vi "Is Connected.vi"(8 "error in (no error)":errorcluster, 11 "FileStream in":refnum<class "FileStream.lvclass">) -> (0 "error out":errorcluster, 2 "Connected":bool, 3 "FileStream out":refnum<class "FileStream.lvclass">)   [LabVIEW 2020, in "Stream.lvlib" / "FileStream.lvclass"]
uses:
  FileStream.lvclass
  FileStream.lvclass/FileStream.ctl
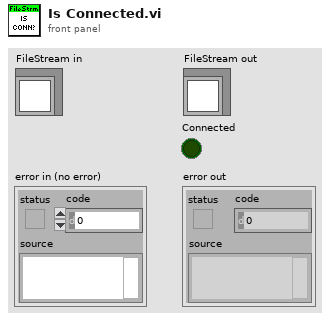
[diagram p1: front panel]
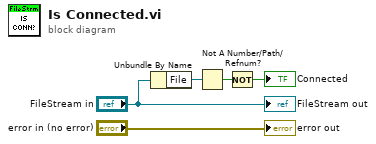
[diagram p0: block diagram]
diagram:
  n1 = Unbundle By Name("FileStream in") -> ("File"=w3:refnum<file>)
  n2 = Not A Number/Path/Refnum?(number/path/refnum=w3) -> (NaN/Path/Refnum?=w2:bool)
  n3 = Not(x=w2) -> (.not. x?=→"Connected":bool)
  "error out" <- "error in (no error)"
  "FileStream out" <- "FileStream in"
